vi "Area_Check Draw Result.vi"(9 "ROI":i32[](array[numeric])=[0, 0, 0, 0], 10 "AreaDataOut":T2(array[cluster]) {"AreaDataOut"."Rectangle"."Rotation" format="%.2f"; "AreaDataOut"."Rectangle"."Left" scale=0.0..1024.0; "AreaDataOut"."Rectangle"."Right" scale=0.0..1024.0}, 11 "Refnum in":T3) -> (0 "error out":errorcluster, 3 "Refnum out":T3)   [LabVIEW 2019]
uses:
  <vilib>/vision/Image Controls.llb/IMAQ Image.ctl
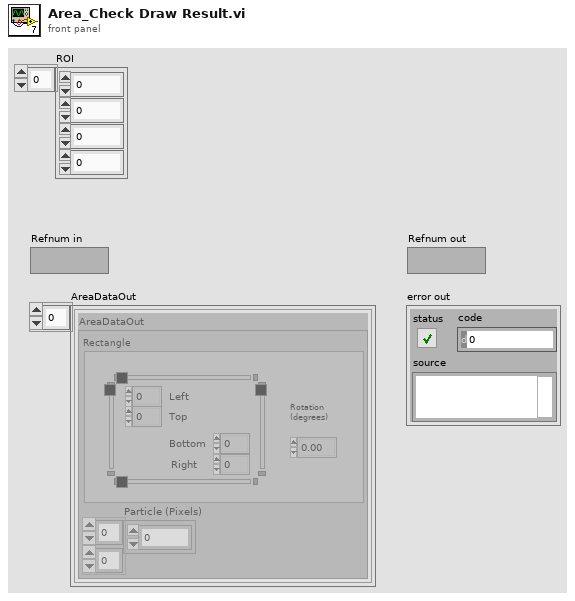
[diagram p1: front panel]
types:
  T1 = typedef "IMAQ Rectangle" = cluster{"Left":i32, "Top":i32, "Right":i32, "Bottom":i32, "Rotation":dbl}
  T2 = cluster{"AreaDataOut":cluster{"Rectangle":T1, "Particle (Pixels)":dbl[][]}}[]
  T3 = typedef "IMAQ Image.ctl" = refnum<image>
  T4 = cluster{"Desired Font (Application)":enum16{"User-specified Font", "Application Font", "System Font", "Dialog Font"}, "[User-specified Font]":cluster{"Font Name":string, "Size":i16, "Strikeout?":bool, "Italic?":bool, "Underline?":bool, "Outline?":bool, "Shadow?":bool, "Bold?":bool, "Rotation Angle":dbl}, "Horizontal Alignment":i16, "Vertical Alignment":i16}
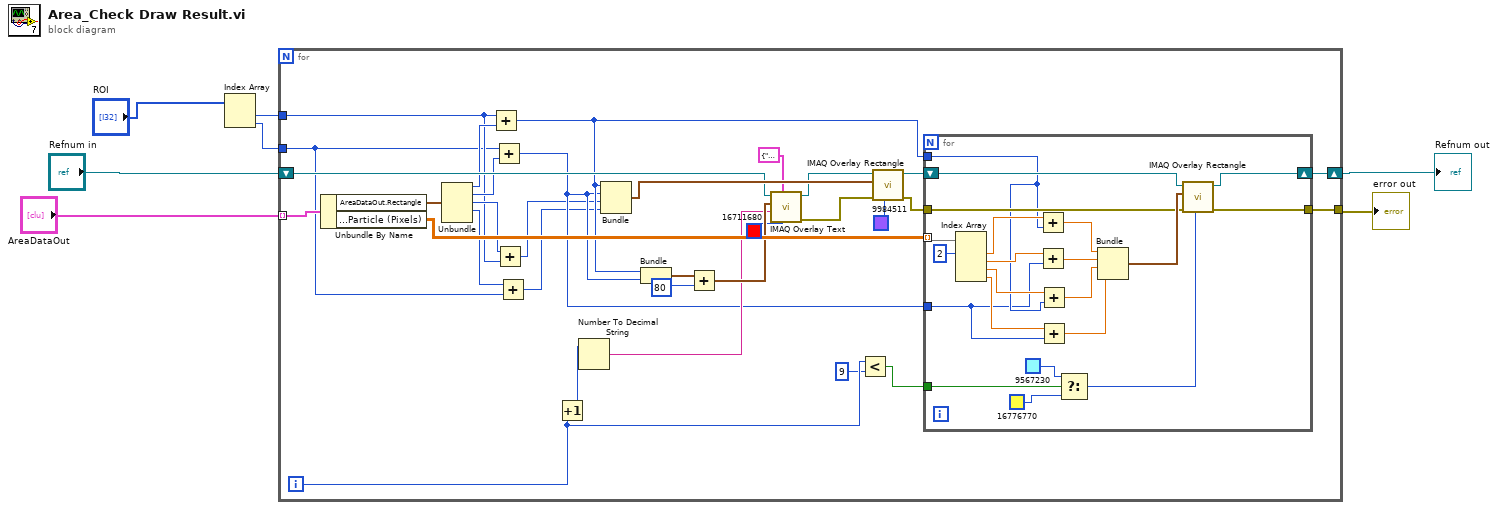
[diagram p0: block diagram]
diagram:
  n1 = Index Array(array="ROI") -> (element #1=w2:i32, element #2=w1:i32)  [unwired: 2 in]
  n2 = for {
    tunnel: "AreaDataOut" -> [w39] mode=indexing
    shift-right: [w21] -> w6
    shift-left: "Refnum in" -> [w31]
    tunnel: [w32] -> w7
    tunnel: w2 -> [w14]
    tunnel: w1 -> [w13]
    i -> [w10]
    n3 = Unbundle By Name(w39) -> ("AreaDataOut.Rectangle"=w38:T1, "AreaDataOut.Particle (Pixels)"=w34:dbl[][])
    n4 = Unbundle(w38) -> ("Left"=w20:i32, "Top"=w18:i32, "Right"=w16:i32, "Bottom"=w15:i32)  [unwired: 1 out]
    n5 = Add(x=w14, y=w20) -> (x+y=w19:i32)
    n6 = Add(x=w13, y=w18) -> (x+y=w17:i32)
    n7 = Add(x=w16, y=w14) -> (x+y=w12:i32)
    n8 = Add(x=w15, y=w13) -> (x+y=w11:i32)
    n9 = Increment(x=w10) -> (x+1=w22:i32)
    n10 = Number To Decimal String(number=w22) -> (decimal integer string=w23:string)  [unwired: 1 in]
    n11 = Bundle(w19, w17, w12, w11) -> (w37:cluster{i32, i32, i32, i32})  [unwired: 1 in]
    n12 = Bundle(w19, w17) -> (w29:cluster{i32, i32})  [unwired: 1 in]
    n13 = Add(x=w29, y=80 ("index")) -> (x+y=w27:cluster{i32, i32})
    n14 = call "IMAQ Overlay Text"("Text Color (black)"=u32 16711680, "Font, Size & Style"=T4 {"Desired Font (Application)"=enum."User-specified Font", "[User-specified Font]"={"Font Name"="", "Size"=96, "Strikeout?"=FALSE, "Italic?"=FALSE, "Underline?"=FALSE, "Outline?"=FALSE, "Shadow?"=FALSE, "Bold?"=FALSE, "Rotation Angle"=0.0}, "Horizontal Alignment"=1, "Vertical Alignment"=0}, "String"=w23, "Origin"=w27, "Image"=w31) -> ("error out"=w25:errorcluster, "Image Out"=w30:T3)  [unwired: 5 in]
    n15 = Less?(x=w10, y=9) -> (x < y?=w8:bool)
    n16 = call "IMAQ Overlay Rectangle"("Color"=u32 9984511, "error in (no error)"=w25, "Rectangle"=w37, "Image"=w30) -> ("error out"=w33:errorcluster, "Image Out"=w35:T3)  [unwired: 6 in]
    n17 = for {
      shift-right: [w57] -> w21
      shift-left: w35 -> [w58]
      tunnel: w34 -> [w60] mode=indexing
      tunnel: w33 -> [w54]
      tunnel: [w55] -> w32
      tunnel: w19 -> [w49]
      tunnel: w17 -> [w48]
      tunnel: w8 -> [w42]
      n18 = Index Array(array=w60, index #1=2 ("index")) -> (element #1=w53:dbl, element #2=w52:dbl, element #3=w51:dbl, element #4=w50:dbl)  [unwired: 3 in]
      n19 = Add(x=w53, y=w49) -> (x+y=w47:dbl)
      n20 = Add(x=w52, y=w48) -> (x+y=w46:dbl)
      n21 = Add(x=w51, y=w49) -> (x+y=w45:dbl)
      n22 = Add(x=w50, y=w48) -> (x+y=w44:dbl)
      n23 = Select(t=u32 9567230 ("Color"), s=w42, f=u32 16776770 ("Color")) -> (s? t:f=w41:u32)
      n24 = Bundle(w47, w46, w45, w44) -> (w56:cluster{dbl, dbl, dbl, dbl})  [unwired: 1 in]
      n25 = call "IMAQ Overlay Rectangle"("Color"=w41, "error in (no error)"=w54, "Rectangle"=w56, "Image"=w58) -> ("error out"=w55:errorcluster, "Image Out"=w57:T3)  [unwired: 6 in]
    }
  }
  "error out" <- w7
  "Refnum out" <- w6
